vi "Write.vi"(8 "error in":errorcluster, 10 "command":string, 11 "VISA resource name":refnum<visa-resource-name>) -> (0 "error out":errorcluster, 3 "VISA resource name out":refnum<visa-resource-name>)   [LabVIEW 2025]
doc: "Write a command to the bridge."
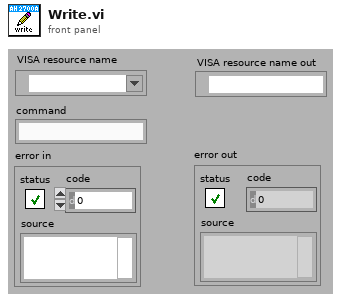
[diagram p1: front panel]
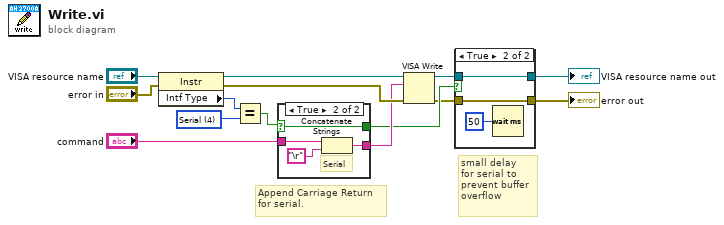
[diagram p0: block diagram]
diagram:
  w10 = u16 4 items=["GPIB"=1, "VXI"=2, "GPIB-VXI"=3, "Serial"=4, "PXI"=5, "TCPIP"=6, "USB"=7, "FireWire"=9] ("Interface Information:Interface Type")
  # "small delay\nfor serial to \nprevent buffer\noverflow"
  # "Append Carriage Return\nfor serial."
  n1 = property class="Instr"(reference="VISA resource name", error in="error in") -> (reference out=w14:refnum<visa-resource-name>, error out=w13:errorcluster, "Intf Type"=w11:u16)
  n2 = Equal?(x=w11, y=w10) -> (x = y?=w7:bool)
  n3 = case shown="True" w7 {
    selector: w7 -> [w15 w17]
    tunnel: "command" -> [w16 w19]
    tunnel: [w16 w18] -> w8
    tunnel: [w15 w17] -> w6
    frame False {
    }
    frame True {
      # "Serial"
      n4 = Concatenate Strings(w19, "\r") -> (w18:string)
    }
  }
  n5 = VISA Write(VISA resource name=w14, write buffer=w8, error in (no error)=w13) -> (VISA resource name out=w4:refnum<visa-resource-name>, error out=w2:errorcluster)  [unwired: 1 out]
  n6 = case shown="True" w6 {
    tunnel: w4 -> [w22 w25]
    tunnel: [w22 w25] -> w3
    tunnel: w2 -> [w21 w24]
    tunnel: [w21 w24] -> w1
    frame False {
    }
    frame True {
      n7 = Wait (ms)(milliseconds to wait=u32 50) -> ()  [unwired: 1 out]
    }
  }
  "VISA resource name out" <- w3
  "error out" <- w1
